vi "InitStaticVIRefs.vi"   [LabVIEW 2019]
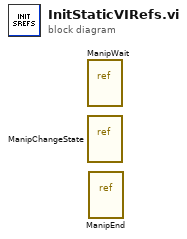
[diagram p0: block diagram]
diagram:
  n1 = vi-ref "ManipWait.vi"() -> ()  [unwired: 1 out]
  n2 = vi-ref "ManipChangeState.vi"() -> ()  [unwired: 1 out]
  n3 = vi-ref "ManipEnd.vi"() -> ()  [unwired: 1 out]
